vi "Configure Voltage Limit.vi"(7 "Slave Address":i32=-1 min=-1 max=30 step=1, 8 "error":errorcluster, 9 "Settle (0 mS)":u32, 10 "Voltage Limit":dbl format="%.4f", 11 "VISA":refnum<visa-resource-name>) -> (0 "error out":errorcluster, 3 "VISA out":refnum<visa-resource-name>)   [LabVIEW 2025, in "TDK-Lambda GEN LAN Series.lvlib"]
doc: "Configure the voltage limit. The power supply output will go to this limit if the load causes Constant-Voltage operation.\n\nThis VI will wait for \"Settle\" milliseconds after setting the limit to allow the output to reach the new setting. If unwired, there will be no delay\n\nNote: The voltage limit must be in the range set by the Under-Voltage Limit and the Over-Voltage Protection settings."
uses:
  <userlib>/TDK-Lambda GEN LAN Series/TDK-Lambda GEN LAN Series.lvlib
panel:
  # "TDK-Lambda Genesys \n LAN\n  DC Power Supplies"
  # "Set the Voltage Limit"
  # "(c) 2019 TDK-Lambda.  ALL RIGHTS RESERVED."
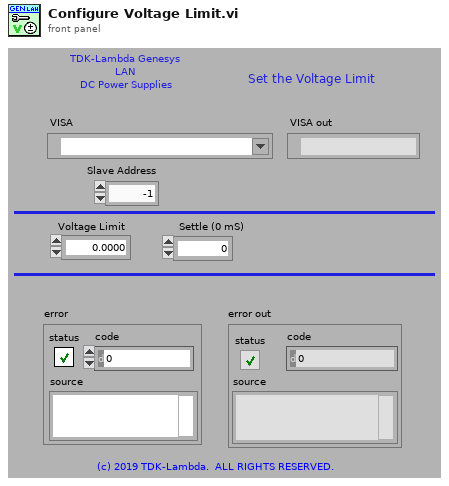
[diagram p1: front panel]
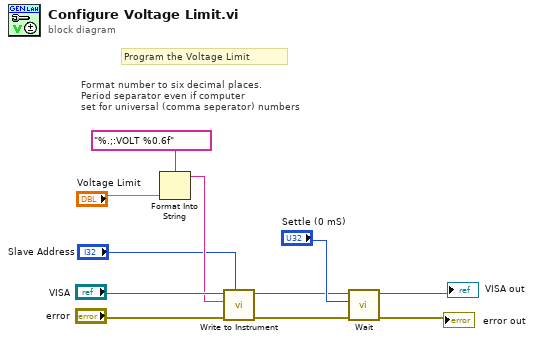
[diagram p0: block diagram]
diagram:
  # "Format number to six decimal places.\nPeriod separator even if computer \nset for universal (comma seperator) numbers"
  # "Program the Voltage Limit"
  n1 = Format Into String(format string="%.;:VOLT %0.6f", "Voltage Limit") -> (resulting string=w4:string)  [unwired: 2 in, 1 out]
  n2 = call <userlib>:"Write to Instrument.vi"("Slave Address"="Slave Address", "error"="error", "Command"=w4, "VISA"="VISA") -> ("error out"=w6:errorcluster, "VISA out"=w7:refnum<visa-resource-name>)  [unwired: 6 in]
  n3 = call <userlib>:"Wait.vi"("error"=w6, "Delay (20 mS)"="Settle (0 mS)", "VISA"=w7) -> ("error out"=→"error out":errorcluster, "VISA out"=→"VISA out":refnum<visa-resource-name>)  [unwired: 7 in]
